vi "Close Shared Memory File.vi"(8 "error in (no error)":errorcluster, 11 "shared memory in":T1) -> (0 "error out":errorcluster, 3 "shared memory out":T1)   [LabVIEW 2013, in "Linux RT IPC.lvlib" / "Shared Memory.lvlib" / "Shared Memory.lvclass"]
doc: "This VI closes the file descriptor that was opened by the Open Shared Memory VI. The file descriptor is a reference to the file that is required to perform the memory mapping process, and closing it will not affect memory that was mapped by the Map Shared Memory VI."
uses:
  Shared Memory.lvclass
  Controls/reference.ctl
  Shared Memory.lvlib
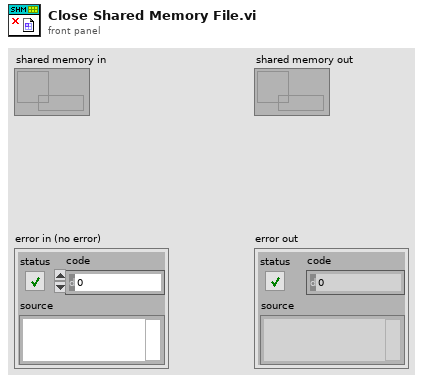
[diagram p1: front panel]
types:
  T1 = typedef "Linux RT IPC.lvlib/Shared Memory.lvlib/reference.ctl" = refnum<data-value>
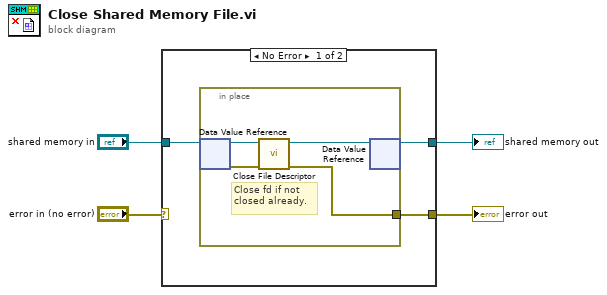
[diagram p0: block diagram]
diagram:
  n1 = case shown="No Error" "error in (no error)" {
    selector: "error in (no error)" -> [_ w13]
    tunnel: "shared memory in" -> [w7 w12]
    tunnel: [w5 w13] -> w2
    tunnel: [w6 w12] -> w1
    frame No Error {
      n2 = in-place {
        in-place-border: [w8] -> w5
        # "Close fd if not closed already."
        n3 = in-place-dvr #1(w7) -> (w11:refnum<class "Shared Memory.lvclass">, w10:errorcluster)
        n4 = call "Close File Descriptor.vi"("error in (no error)"=w10, "Shared Memory in"=w11) -> ("error out"=w8:errorcluster, "Shared Memory out"=w9:refnum<class "Shared Memory.lvclass">)  [unwired: 8 in]
        n5 = in-place-dvr #1(w9) -> (w6:T1)  [unwired: 1 out]
      }
    }
    frame Error {
    }
  }
  "error out" <- w2
  "shared memory out" <- w1
